vi "MBtcp-OpenWriteClose.vi"(4 "RegisterType":T1="Input", 5 "Slave ID":u8=255 format="%.0x", 6 "Timeout (900)":i32=900, 8 "error in (no error)":errorcluster, 9 "Values":u16[](array[numeric]), 10 "RegisterAddr":u16, 11 "IP Address(:port)":string) -> (0 "error out":errorcluster)   [LabVIEW 2018]
uses:
  RegisterTypes.ctl
  <vilib>/Plasmionique/MB Master/MB_Master_TCP/MB_Master_TCP.lvclass
  C:/Program Files/National Instruments/LabVIEW 2018/vi.lib/Plasmionique/MB Master/MB_Master/MB_Master.lvclass
  <vilib>/Plasmionique/MB Master/MB Master.lvlib
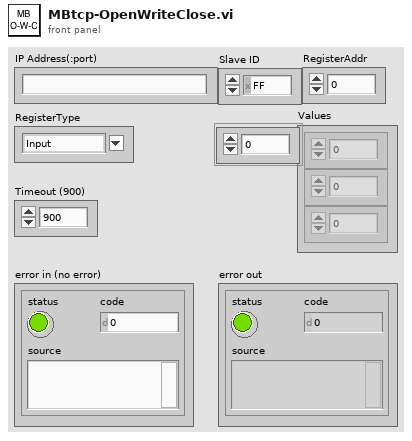
[diagram p1: front panel]
types:
  T1 = typedef "RegisterTypes.ctl" = string
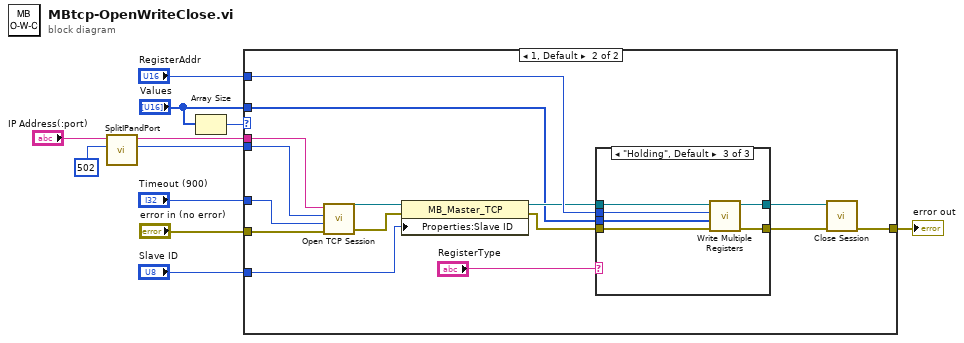
[diagram p0: block diagram]
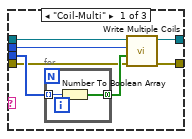
[diagram p3: hidden frame]
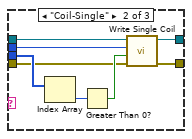
[diagram p4: hidden frame]
diagram:
  n1 = call "SplitIPandPort.vi"("defaultPort(10001)"=u16 502, "IP:Port"="IP Address(:port)") -> ("Port"=w2:u16, "IP"=w4:string)  [unwired: 8 in]
  n2 = Array Size(array="Values") -> (size(s)=w6:i32)
  n3 = case shown="1, Default" w6 {
    tunnel: [w12 w27] -> w11
    tunnel: "RegisterAddr" -> [_ w26]
    tunnel: w4 -> [_ w25]
    tunnel: "error in (no error)" -> [w12 w24]
    tunnel: "Timeout (900)" -> [_ w23]
    tunnel: "Slave ID" -> [_ w16]
    tunnel: "Values" -> [_ w14]
    tunnel: w2 -> [_ w13]
    frame 0 {
    }
    frame 1, Default {
      n4 = call <vilib>:"Open TCP Session.vi"("error in (no error)"=w24, "Timeout (10000)"=w23, "Port (502)"=w13, "IP Address"=w25) -> ("error out"=w18:errorcluster, "MB_TCP session"=w20:refnum<class "MB_Master_TCP.lvclass">)  [unwired: 6 in]
      n5 = property class="MB_Master_TCP"(reference=w20, error in=w18, "Properties:Slave ID"=w16) -> (reference out=w19:refnum<class "MB_Master_TCP.lvclass">, error out=w17:errorcluster)
      n6 = case shown="\"Holding\", Default" "RegisterType" {
        tunnel: w26 -> [w29 w41 w50]
        tunnel: [w32 w43 w49] -> w22
        tunnel: [w33 w44 w48] -> w21
        tunnel: w19 -> [w31 w42 w47]
        tunnel: w17 -> [w28 w37 w46]
        tunnel: w14 -> [w30 w39 w45]
        frame "Coil-Multi" {
          n7 = for {
            tunnel: w30 -> [w36] mode=indexing
            tunnel: [w35] -> w34 mode=concatenating
            n8 = Number To Boolean Array(number=w36) -> (Boolean array=w35:bool[])
          }
          n9 = call <vilib>:"Write Multiple Coils.vi"("error in (no error)"=w28, "values"=w34, "starting address"=w29, "MB session in"=w31) -> ("error out"=w32:errorcluster, "MB session out"=w33:refnum<class "MB_Master_TCP.lvclass">)  [unwired: 6 in]
        }
        frame "Coil-Single" {
          n10 = Index Array(array=w39) -> (element=w38:u16)  [unwired: 1 in]
          n11 = Greater Than 0?(x=w38) -> (x > 0?=w40:bool)
          n12 = call <vilib>:"Write Single Coil.vi"("error in (no error)"=w37, "value"=w40, "address"=w41, "MB session in"=w42) -> ("error out"=w43:errorcluster, "MB session out"=w44:refnum<class "MB_Master_TCP.lvclass">)  [unwired: 6 in]
        }
        frame "Holding", Default {
          n13 = call <vilib>:"Write Multiple Registers.vi"("error in (no error)"=w46, "values"=w45, "starting address"=w50, "MB session in"=w47) -> ("error out"=w49:errorcluster, "MB session out"=w48:refnum<class "MB_Master_TCP.lvclass">)  [unwired: 6 in]
        }
      }
      n14 = call-dynamic "Close Session.vi"("error in (no error)"=w22, "MB TCP session"=w21) -> ("error out"=w27:errorcluster)  [unwired: 9 in]
    }
  }
  "error out" <- w11
